vi "DeserializeAndRevert.vi"(11 "U16 input":u16) -> (3 "10bit output":bool[](array[boolean]))   [LabVIEW 2012]
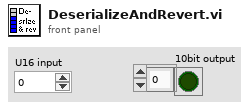
[diagram p1: front panel]
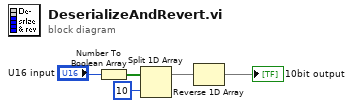
[diagram p0: block diagram]
diagram:
  n1 = Number To Boolean Array(number="U16 input") -> (Boolean array=w4:bool[])
  n2 = Split 1D Array(array=w4, index=10) -> (first subarray=w2:bool[])  [unwired: 1 out]
  n3 = Reverse 1D Array(array=w2) -> (reversed array=→"10bit output":bool[])
